vi "Open Device (serial number).vi"(8 "error in (no error)":errorcluster, 10 "Device Serial Number":string) -> (0 "error out":errorcluster, 3 "Handle":u32)   [LabVIEW 2019, in "D2XX-lv.lvlib"]
uses:
  D2XX-lv.lvlib
  D2XX_Functions_7.0/D2XX.lvlib
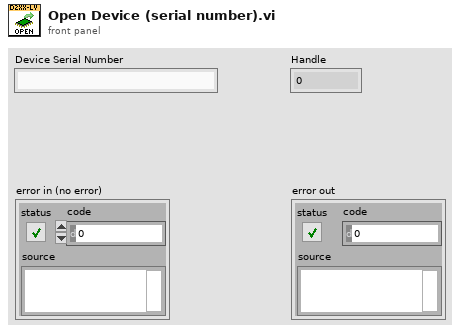
[diagram p1: front panel]
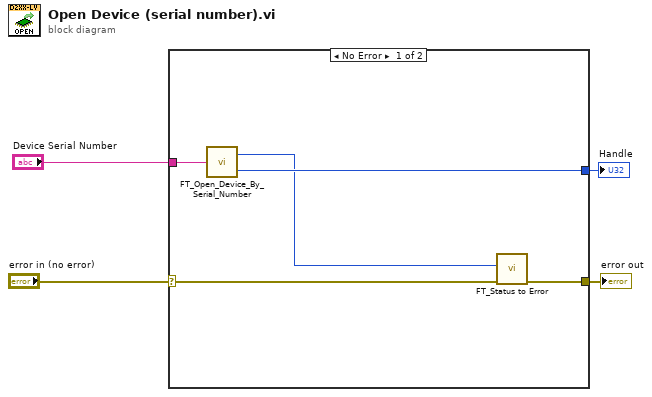
[diagram p0: block diagram]
diagram:
  n1 = case shown="No Error" "error in (no error)" {
    selector: "error in (no error)" -> [w9 w10]
    tunnel: [w8 w10] -> w3
    tunnel: "Device Serial Number" -> [w7 _]
    tunnel: [w6 _] -> w1
    frame No Error {
      n2 = call "FT_Open_Device_By_Serial_Number.vi"("Device Serial Number"=w7) -> ("FT_Status"=w5:u32, "Handle"=w6:u32)
      n3 = call "FT_Status to Error.vi"("error in (no error)"=w9, "FT_Status"=w5) -> ("error out"=w8:errorcluster)  [unwired: 9 in]
    }
    frame Error {
    }
  }
  "error out" <- w3
  "Handle" <- w1
